vi "PH_GUI.Manager Path.vi"(1 "i ref in":refnum<vi>) -> (0 "GUI Manager Path":path)   [LabVIEW 2014, in "PH_Common.lvlib"]
doc: "This VI sets the path to get or to set the position of the GUI panel to a xml-file."
uses:
  PH_Common.lvlib
  CS_Core/CSSystem/CSSystemLib/CSSystemLib.lvlib
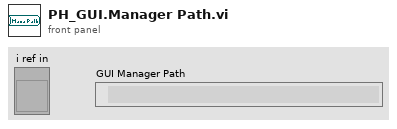
[diagram p1: front panel]
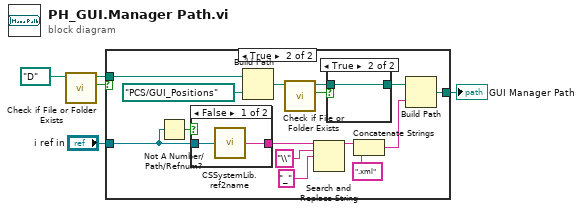
[diagram p0: block diagram]
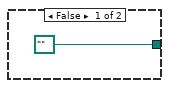
[diagram p2: hidden frame]
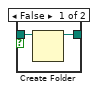
[diagram p3: hidden frame]
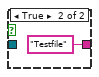
[diagram p4: hidden frame]
diagram:
  n1 = call <vilib>:"Check if File or Folder Exists.vi"("path"=path "D:/") -> ("file or folder exists?"=w2:bool, "dup path"=w1:path)  [unwired: 8 in, 1 out]
  n2 = case shown="True" w2 {
    tunnel: [path "" ("appended path") w15] -> w5
    tunnel: "i ref in" -> [_ w14]
    tunnel: w1 -> [_ w12]
    frame False {
    }
    frame True {
      n3 = Not A Number/Path/Refnum?(number/path/refnum=w14) -> (NaN/Path/Refnum?=w13:bool)
      n4 = case shown="False" w13 {
        tunnel: [w26 "Testfile" ("name")] -> w18
        tunnel: w14 -> [w25 _]
        frame False {
          n5 = call "CSSystemLib.ref2name.vi"("obj refnum"=w25) -> ("name"=w26:string)
        }
        frame True {
        }
      }
      n6 = Build Path(base path=w12, name or relative path=path "PCS/GUI_Positions" ("path")) -> (appended path=w10:path)
      n7 = call <vilib>:"Check if File or Folder Exists.vi"("path"=w10) -> ("file or folder exists?"=w9:bool, "dup path"=w8:path)  [unwired: 8 in, 1 out]
      n8 = Search and Replace String(input string=w18, search string="\\", replace string="_" ("replace string (\"\")")) -> (result string=w19:string)  [unwired: 5 in, 3 out]
      n9 = case shown="True" w9 {
        tunnel: w8 -> [w23 w24]
        tunnel: [w22 w24] -> w7
        frame False {
          n10 = Create Folder(path (use dialog)=w23) -> (created path=w22:path)  [unwired: 2 in, 2 out]
        }
        frame True {
        }
      }
      n11 = Concatenate Strings(w19, ".xml" ("string")) -> (w16:string)
      n12 = Build Path(base path=w7, name or relative path=w16) -> (appended path=w15:path)
    }
  }
  "GUI Manager Path" <- w5
